vi "Set Timeouts.vi"(8 "error in (no error)":errorcluster, 9 "write operation timeout (ms)":i32=5000, 10 "read operation timeout (ms)":i32=5000, 11 "Modbus master in":refnum<class "Network Master.lvclass">) -> (0 "error out":errorcluster, 3 "Modbus master out":refnum<class "Network Master.lvclass">)   [LabVIEW 2021, in "Modbus Master.lvclass"]
doc: "Sets both read and write operation timeouts on a Modbus slave."
uses:
  Modbus Master.lvclass
  Modbus Master.lvclass/Modbus Master.ctl
  Transmission Data Unit/Transmission Data Unit.lvclass
  Network Protocol/Network Master/Network Master.lvclass
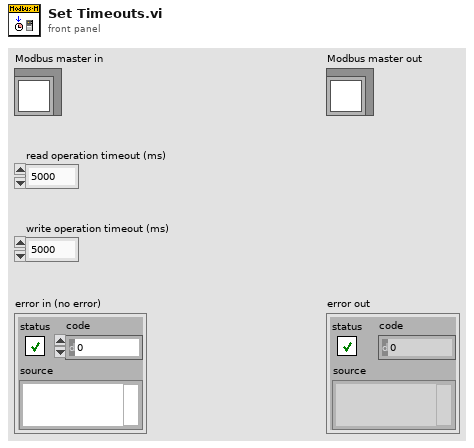
[diagram p1: front panel]
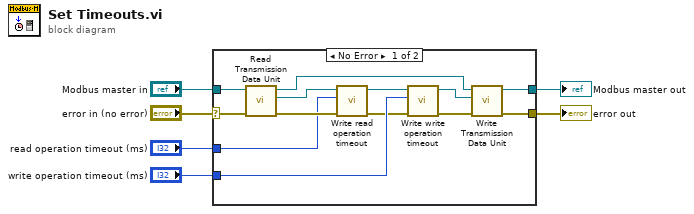
[diagram p0: block diagram]
diagram:
  n1 = case shown="No Error" "error in (no error)" {
    selector: "error in (no error)" -> [w8 w21]
    tunnel: "write operation timeout (ms)" -> [w15 _]
    tunnel: "read operation timeout (ms)" -> [w14 _]
    tunnel: [w11 w20] -> w4
    tunnel: [w10 w21] -> w3
    tunnel: "Modbus master in" -> [w9 w20]
    frame No Error {
      n2 = call "Read Transmission Data Unit.vi"("error in (no error)"=w8, "Network Master in"=w9) -> ("error out"=w18:errorcluster, "Transmission Data Unit"=w19:refnum<class "Transmission Data Unit.lvclass">, "Network Master out"=w7:refnum<class "Network Master.lvclass">)  [unwired: 7 in]
      n3 = call "Write read operation timeout.vi"("error in (no error)"=w18, "read operation timeout"=w14, "transmission data unit in"=w19) -> ("error out"=w13:errorcluster, "transmission data unit out"=w16:refnum<class "Transmission Data Unit.lvclass">)  [unwired: 7 in]
      n4 = call "Write write operation timeout.vi"("error in (no error)"=w13, "write operation timeout"=w15, "transmission data unit in"=w16) -> ("error out"=w12:errorcluster, "transmission data unit out"=w17:refnum<class "Transmission Data Unit.lvclass">)  [unwired: 7 in]
      n5 = call "Write Transmission Data Unit.vi"("error in (no error)"=w12, "Transmission Data Unit"=w17, "Network Master in"=w7) -> ("error out"=w10:errorcluster, "Network Master out"=w11:refnum<class "Network Master.lvclass">)  [unwired: 7 in]
    }
    frame Error {
    }
  }
  "error out" <- w3
  "Modbus master out" <- w4
